vi "attck_din.vi"(9 "balls":T7[](array[typedef]), 10 "IA State":T1={"our_robots"=[], "enemy_robots"=[], "balls"=[], "geometry"={"field_length"=0, "field_width"=0, "goal_width"=0, "goal_depth"=0, "center_circle_radius"=0, "defense_width"=0, "defense_depth"=0, "free_kick_from_defense_dist"=0, "penalty_spot_from_field_line_dist"=0, "penalty_line_from_spot_dist"=0, "half_moon_depth"=0, "half_moon_width"=0}, "IA Judge"={"stage"="", "command"="", "our_goalie_id"=0.0, "enemy_goalie_id"=0.0, "command enum"=enum."Halt", "Time"=enum."Azul"}, "Received Timestamp"=timestamp(0 s since 1904-01-01), "Events"={"Touch"=FALSE, "id touch"=0.0, "Ball out of \nVision"=FALSE, "Ball inside \nGoalie area"=FALSE, "Robot not responding"=FALSE, "Robots responding status"=[1.0, 1.0, 1.0, 1.0, 1.0, 1.0], "Enemy Ball \nPossession"=FALSE, "Id ini Possession"=0.0, "Ball Possesion"=FALSE, "Id Possesion"=0.0, "Ball at\nour goal side"=FALSE, "Ball at\ntouchline"=FALSE, "Ball at\nenemy goal side"=FALSE}}, 11 "Robot in":T2) -> (3 "Robot out":T2)   [LabVIEW 2018]
uses:
  Core/AI Robot.ctl
  Functions Enum.ctl
  AttackerStates.ctl
  Path Planning/RRT/PathDests.ctl
  Path Planning/RRT/PathDest.ctl
  Core/AI Ball.ctl
  Core/AI Input.ctl
  Core/Field Size.ctl
  Core/AI Judge.ctl
  Command Enum.ctl
  Util/Events/Events.ctl
  <vilib>/Analysis/_algsub.llb/Real Vector Norm.vi
  <vilib>/Analysis/NI_AALPro.lvlib
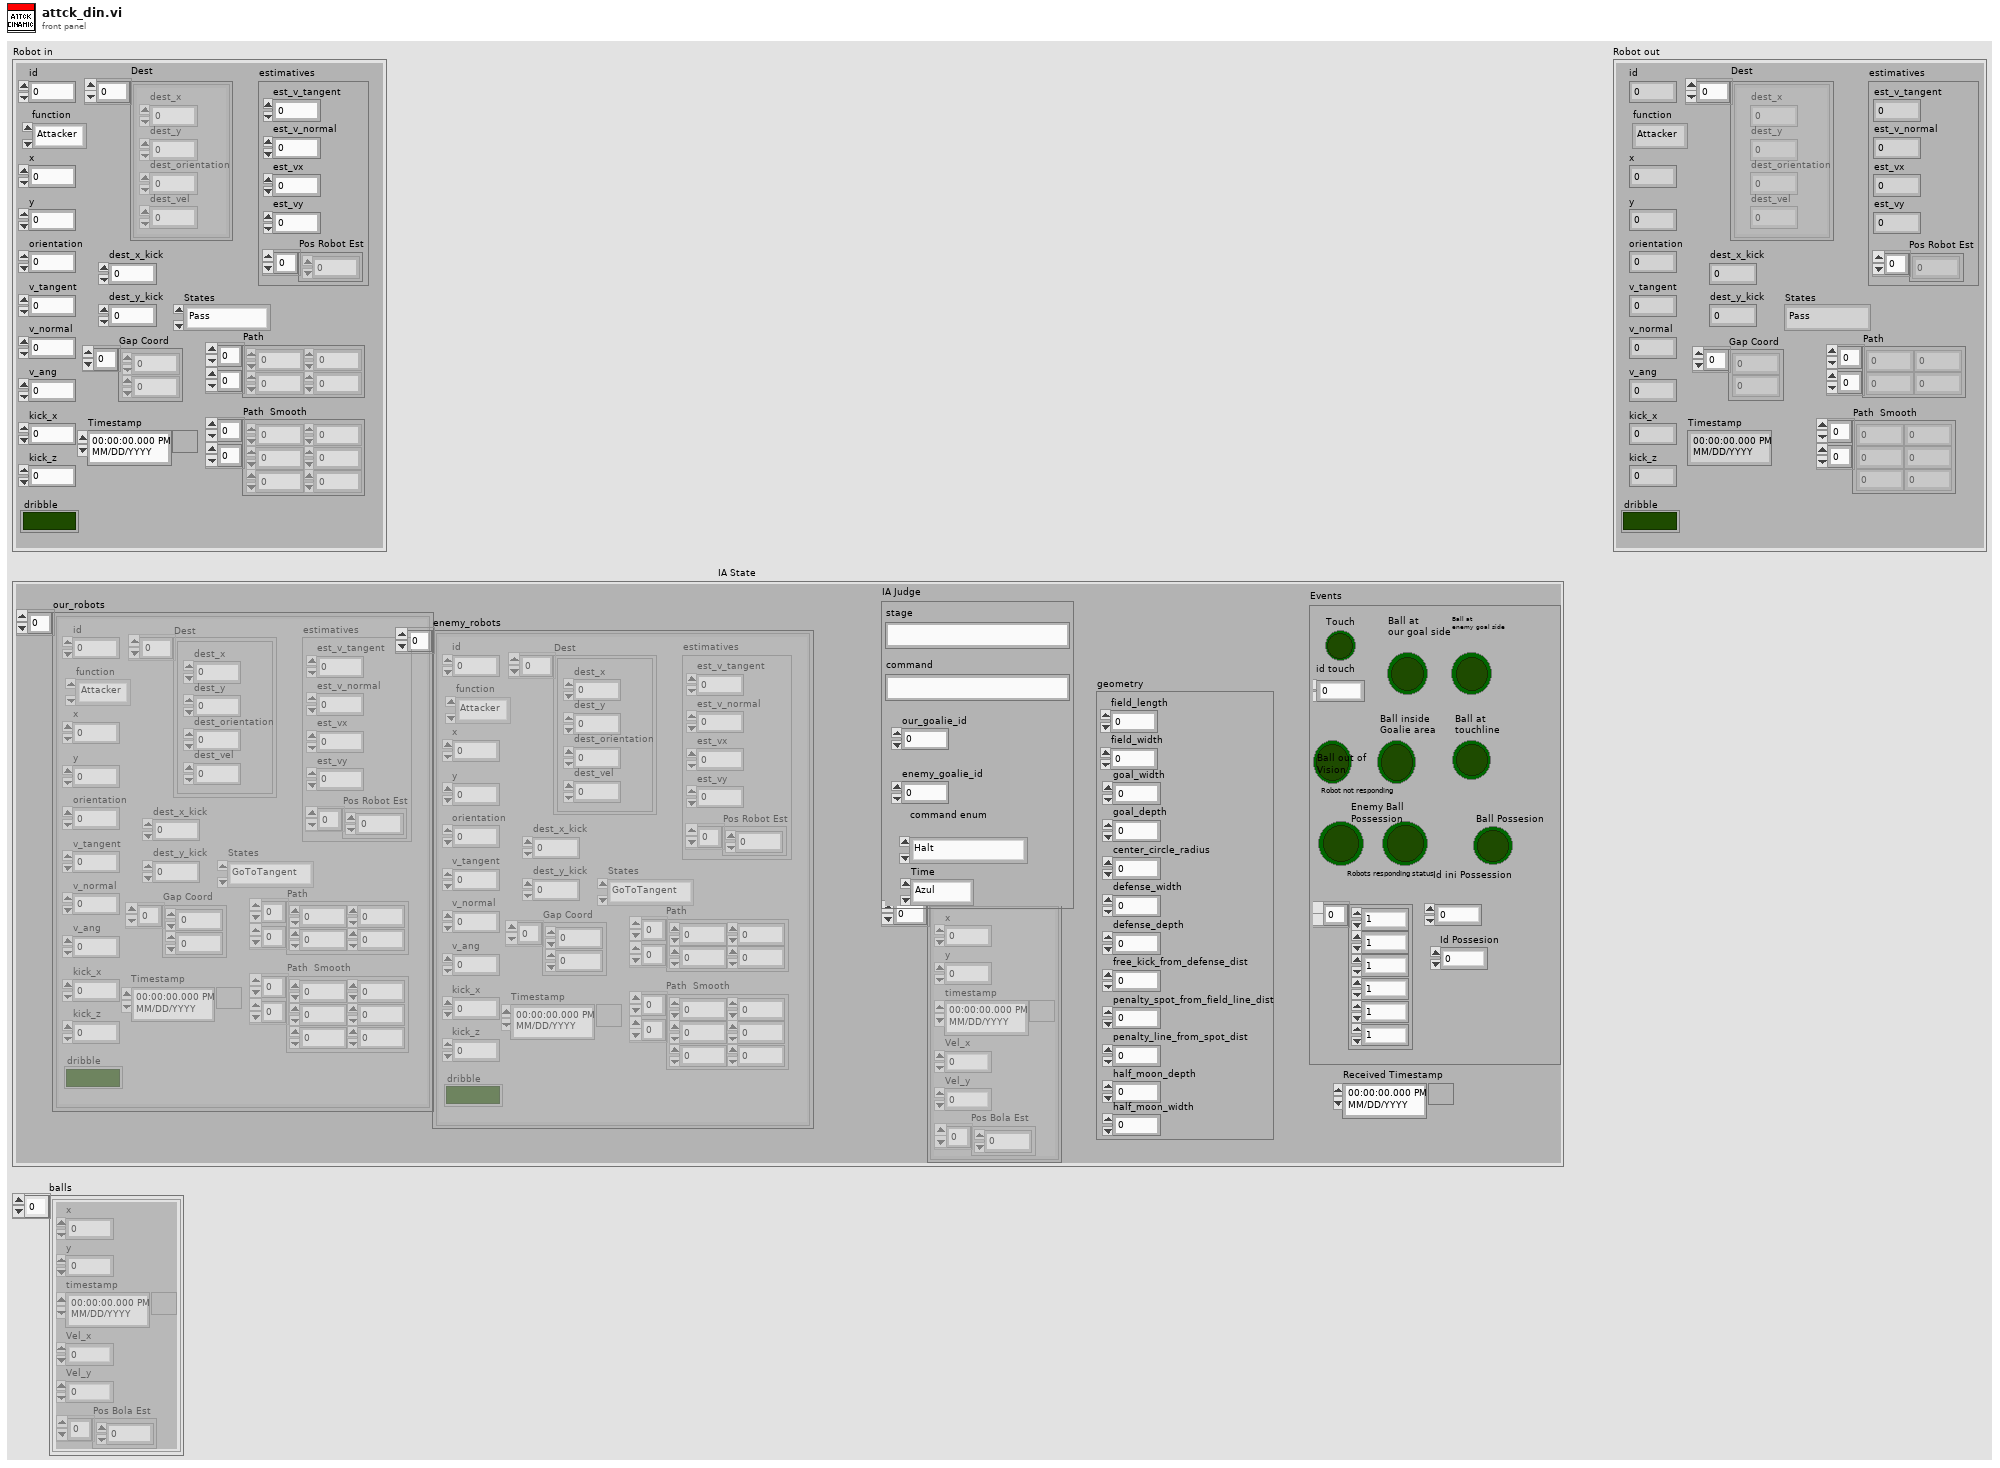
[diagram p1: front panel]
types:
  T1 = typedef "AI Input.ctl" = cluster{"our_robots":T2[], "enemy_robots":T2[], "balls":T7[], "geometry":T8, "IA Judge":T9, "Received Timestamp":timestamp, "Events":T11}
  T2 = typedef "AI Robot.ctl" = cluster{"id":u32, "function":T3, "x":dbl, "y":dbl, "orientation":dbl, "v_tangent":dbl, "v_normal":dbl, "v_ang":dbl, "kick_x":dbl, "kick_z":dbl, "dribble":bool, "Timestamp":timestamp, "estimatives":cluster{"est_v_tangent":dbl, "est_v_normal":dbl, "est_vx":dbl, "est_vy":dbl, "Pos Robot Est":dbl[]}, "dest_x_kick":dbl, "dest_y_kick":dbl, "Gap Coord":dbl[], "States":T4, "Path ":dbl[][], "Path  Smooth":dbl[][], "Dest":T5}
  T3 = typedef "Functions Enum.ctl" = enum16{"Attacker", "Goalie", "Defender", "Striker", "Goto 0", "Dummy", "Kicker", "ZigZag"}
  T4 = typedef "AttackerStates.ctl" = enum16{"Pass", "GoToTangent", "BallGetting", "GoToKick", "Rotate anti-clockwise", "Rotate Clockwise", ""}
  T5 = typedef "PathDests.ctl" = T6[]
  T6 = typedef "PathDest.ctl" = cluster{"dest_x":dbl, "dest_y":dbl, "dest_orientation":dbl, "dest_vel":dbl}
  T7 = typedef "AI Ball.ctl" = cluster{"x":dbl, "y":dbl, "timestamp":timestamp, "Vel_x":dbl, "Vel_y":dbl, "Pos Bola Est":dbl[]}
  T8 = typedef "Field Size.ctl" = cluster{"field_length":u32, "field_width":u32, "goal_width":u32, "goal_depth":u32, "center_circle_radius":u32, "defense_width":u32, "defense_depth":u32, "free_kick_from_defense_dist":u32, "penalty_spot_from_field_line_dist":u32, "penalty_line_from_spot_dist":u32, "half_moon_depth":u32, "half_moon_width":u32}
  T9 = typedef "AI Judge.ctl" = cluster{"stage":string, "command":string, "our_goalie_id":dbl, "enemy_goalie_id":dbl, "command enum":T10, "Time":enum16{"Azul", "Amarelo"}}
  T10 = typedef "Command Enum.ctl" = enum16{"Halt", "Stop", "Force Start", "PKA Normal Start", "Prepare Kickoff Ally", "PKE Normal Start", "Prepare Kickoff Enemy", "Prepare Penalty Ally", "PPA Normal Start", "Prepare Penalty Enemy", "PPE Normal Start", "Ball Placement Enemy Up", "Ball Placement Enemy Down", "Ball Placement Ally Up", "Ball Placement Ally Mid", "Ball Placement Ally Down", "Indirect Free Enemy", "Indirect Free Ally", "Timeout Enemy", "Timeout Ally", "Goal Enemy", "Goal Ally", "Normal Half Time", "Extra Time Break", "Extra Half Time", "None", "Post Game"}
  T11 = typedef "Events.ctl" = cluster{"Touch":bool, "id touch":dbl, "Ball out of \nVision":bool, "Ball inside \nGoalie area":bool, "Robot not responding":bool, "Robots responding status":dbl[], "Enemy Ball \nPossession":bool, "Id ini Possession":dbl, "Ball Possesion":bool, "Id Possesion":dbl, "Ball at\nour goal side":bool, "Ball at\ntouchline":bool, "Ball at\nenemy goal side":bool}
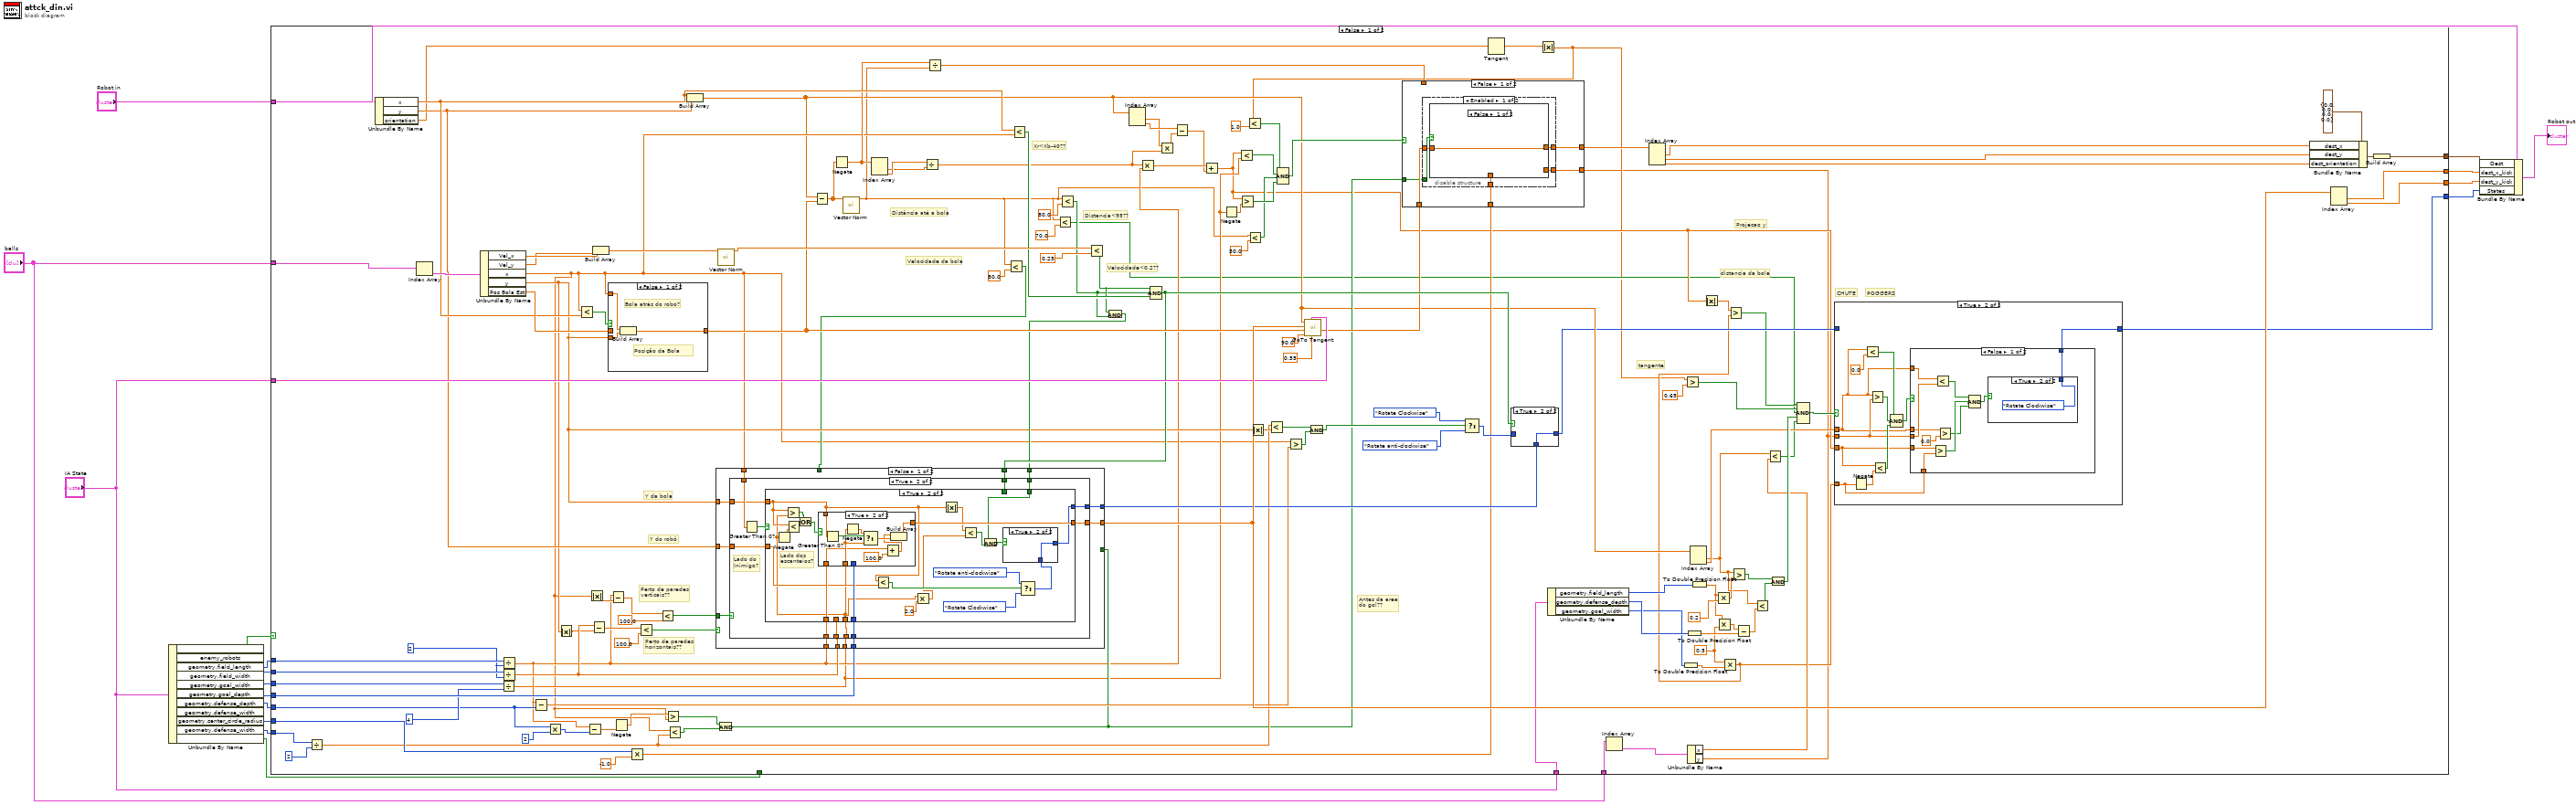
[diagram p0: block diagram]
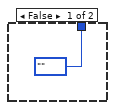
[diagram p3: hidden frame]
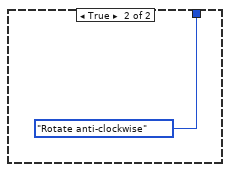
[diagram p4: hidden frame]
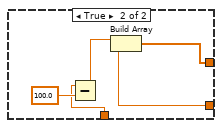
[diagram p5: hidden frame]
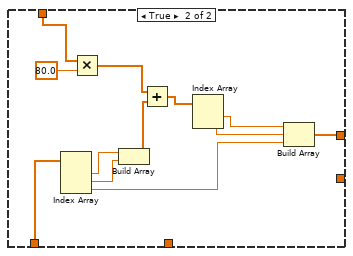
[diagram p7: hidden frame]
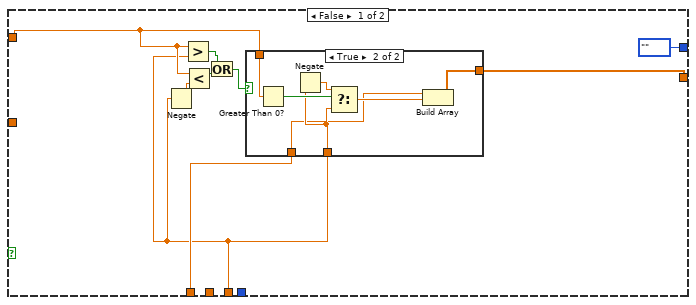
[diagram p10: hidden frame]
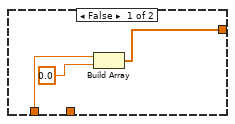
[diagram p11: hidden frame]
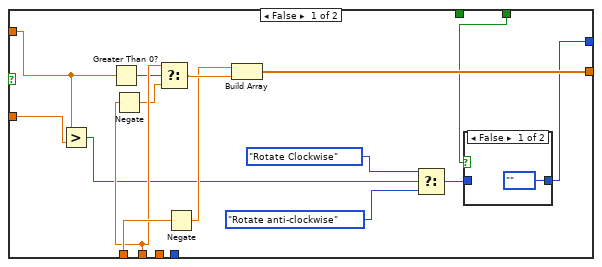
[diagram p12: hidden frame]
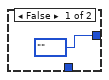
[diagram p14: hidden frame]
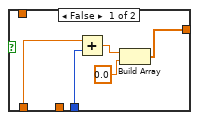
[diagram p15: hidden frame]
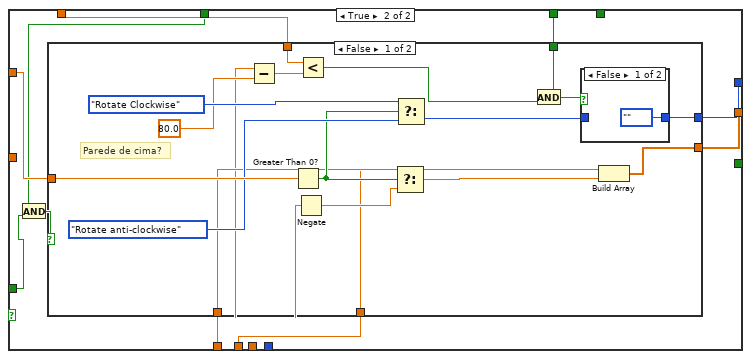
[diagram p16: hidden frame]
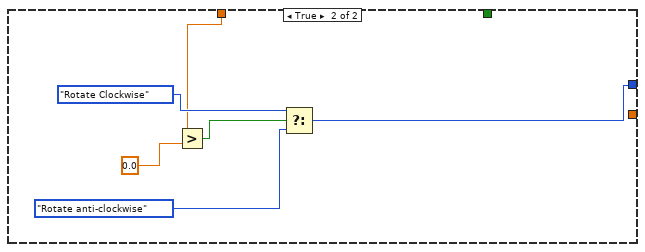
[diagram p18: hidden frame]
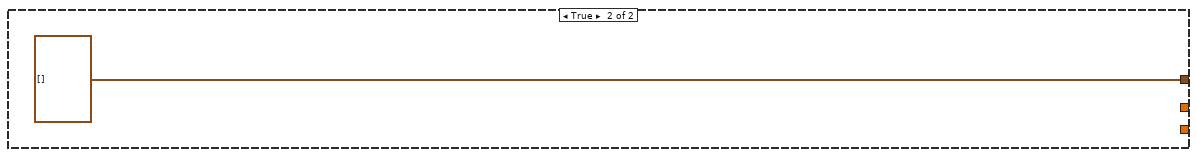
[diagram p19: hidden frame]
diagram:
  n1 = Unbundle By Name("IA State") -> ("Events.Ball out of \nVision"=w6:bool, "geometry.field_length"=w13:u32, "geometry.field_width"=w14:u32, "geometry.goal_width"=w15:u32, "geometry.goal_depth"=w9:u32, "geometry.defense_depth"=w7:u32, "geometry.center_circle_radius"=w4:u32, "geometry.defense_width"=w8:u32, "Events.Ball inside \nGoalie area"=w5:bool)  [unwired: 2 out]
  n2 = case shown="False" w6 {
    tunnel: [w151 _] -> w17
    tunnel: [w150 _] -> w16
    tunnel: w15 -> [w148 _]
    tunnel: "IA State" -> [w147 _]
    tunnel: w14 -> [w143 _]
    tunnel: w13 -> [w142 _]
    tunnel: "Robot in" -> [w141 _]
    tunnel: "balls" -> [w140 _]
    tunnel: [w137 T6[] []] -> w11
    tunnel: w9 -> [w136 _]
    tunnel: w8 -> [w135 _]
    tunnel: w7 -> [w96 _]
    tunnel: w5 -> [_ _]
    tunnel: w4 -> [w90 _]
    tunnel: "IA State" -> [w56 _]
    tunnel: "balls" -> [w58 _]
    tunnel: [w30 _] -> w1
    frame False {
      w36 = 0.5 ("y")
      w130 = u32 2 ("y")
      # "Y do robô"
      # "Y da bola"
      # "distancia da bola"
      # "tangente"
      # "Projecao y"
      # "POGGERS"
      # "CHUTE"
      # "Antes da area \ndo gol??"
      # "Perto de paredes \nverticais??"
      # "Perto de paredes \nhorizontais??"
      # "Velocidade<0,2??"
      # "Distancia<95??"
      # "Xr<Xb-40??"
      # "Velocidade da bola"
      # "Distância até a bola"
      n3 = Divide(x=w135, y=u32 2) -> (x/y=w86:dbl)
      n4 = Unbundle By Name(w141) -> ("x"=w113:dbl, "y"=w100:dbl, "orientation"=w51:dbl)
      n5 = Index Array(array=w140) -> (element=w133:T7)  [unwired: 1 in]
      n6 = Unbundle By Name(w133) -> ("Vel_x"=w123:dbl, "Vel_y"=w122:dbl, "x"=w59:dbl, "y"=w93:dbl, "Pos Bola Est"=w114:dbl[])
      n7 = Divide(x=w148, y=u32 4) -> (x/y=w67:dbl)
      n8 = Divide(x=w142, y=w130) -> (x/y=w75:dbl)
      n9 = Divide(x=w143, y=w130) -> (x/y=w117:dbl)
      n10 = Subtract(x=w75, y=w96) -> (x-y=w104:dbl)
      n11 = Multiply(x=w96, y=u32 2) -> (x*y=w95:u32)
      n12 = Absolute Value(x=w93) -> (abs(x)=w85:dbl)
      n13 = Less?(x=w59, y=w113) -> (x < y?=w116:bool)
      n14 = Subtract(x=w75, y=w95) -> (x-y=w94:dbl)
      n15 = Absolute Value(x=w59) -> (abs(x)=w129:dbl)
      n16 = Subtract(x=w117, y=w85) -> (x-y=w127:dbl)
      n17 = Build Array(w123, w122) -> (w121:dbl[])
      n18 = case shown="False" w116 {
        tunnel: [w209 w212] -> w115
        tunnel: w114 -> [_ w212]
        tunnel: w59 -> [w211 _]
        tunnel: w93 -> [w210 _]
        frame False {
          # "Bola atrás do robo?"
          # "Posição da Bola"
          n19 = Build Array(w211, w210) -> (w209:dbl[])
        }
        frame True {
          # "Posição futura da bola"
          # "Bola atrás do robo?"
        }
      }
      n20 = Subtract(x=w75, y=w129) -> (x-y=w128:dbl)
      n21 = Negate(x=w94) -> (-x=w92:dbl)
      n22 = Multiply(x=w90, y=-1.0) -> (x*y=w87:dbl)
      n23 = Less?(x=w127, y=100.0) -> (x < y?=w126:bool)
      n24 = Less?(x=w128, y=100.0) -> (x < y?=w125:bool)
      n25 = Greater?(x=w92, y=w59) -> (0:w83:bool)
      n26 = Less?(x=w59, y=w86) -> (x < y?=w84:bool)
      n27 = Build Array(w113, w100) -> (w53:dbl[])
      n28 = call-poly <vilib>:"Vector Norm.vi"("Input Vector"=w121) -> ("norm"=w119:dbl)  [unwired: 9 in, 1 out]
      n29 = And(x=w83, y=w84) -> (x .and. y?=w82:bool)
      n30 = Subtract(x=w53, y=w115) -> (x-y=w78:dbl[])
      n31 = Negate(x=w78) -> (-x=w61:dbl[])
      n32 = call-poly <vilib>:"Vector Norm.vi"("Input Vector"=w78) -> ("norm"=w22:dbl)  [unwired: 9 in, 1 out]
      n33 = Index Array(array=w61) -> (element #1=w76:dbl, element #2=w77:dbl)  [unwired: 2 in]
      n34 = Divide(x=w77, y=w76) -> (x/y=w71:dbl)
      n35 = Divide(x=w61, y=w22) -> (x/y=w60:dbl[])
      n36 = Less?(x=w22, y=80.0) -> (x < y?=w79:bool)
      n37 = Less?(x=w113, y=w59) -> (x < y?=w112:bool)
      n38 = Less?(x=w22, y=70.0) -> (x < y?=w23:bool)
      n39 = Less?(x=w22, y=80.0) -> (x < y?=w39:bool)
      n40 = Less?(x=w119, y=0.25) -> (x < y?=w99:bool)
      n41 = And(x=w99, y=w39) -> (x .and. y?=w98:bool)
      n42 = Index Array(array=w53) -> (element #1=w72:dbl, element #2=w74:dbl)  [unwired: 2 in]
      n43 = Multiply(x=w71, y=w75) -> (x*y=w73:dbl)
      n44 = Compound Arithmetic op=AND(w99, w39, w112) -> (w107:bool)
      n45 = case shown="False" w126 {
        tunnel: w93 -> [w222 w319]
        tunnel: w117 -> [w213 w313]
        tunnel: [w221 w318] -> w149
        tunnel: w125 -> [w224 w311]
        tunnel: w59 -> [w223 w315]
        tunnel: w75 -> [w220 w314]
        tunnel: w67 -> [w216 _]
        tunnel: w107 -> [w219 w316]
        tunnel: [w218 w317] -> w106
        tunnel: w136 -> [w217 _]
        tunnel: w100 -> [w215 _]
        tunnel: w98 -> [w214 _]
        tunnel: w82 -> [_ _]
        tunnel: w79 -> [_ w310]
        frame False {
          n46 = case shown="True" w224 {
            tunnel: w223 -> [_ w254]
            tunnel: w222 -> [w231 w253]
            tunnel: [w232 w252] -> w221
            tunnel: w220 -> [w233 w251]
            tunnel: w219 -> [_ w250]
            tunnel: [AttackerStates."" ("States") w249] -> w218
            tunnel: w217 -> [_ w248]
            tunnel: w213 -> [_ w247]
            tunnel: w216 -> [w229 w246]
            tunnel: w215 -> [_ w245]
            tunnel: w214 -> [_ w244]
            frame False {
              n47 = Negate(x=w229) -> (-x=w228:dbl)
              n48 = Greater?(x=w231, y=w229) -> (0:w225:bool)
              n49 = Less?(x=w231, y=w228) -> (x < y?=w226:bool)
              n50 = Or(x=w225, y=w226) -> (x .or. y?=w227:bool)
              n51 = case shown="True" w227 {
                tunnel: w233 -> [w235 w238]
                tunnel: [w236 w237] -> w232
                tunnel: w231 -> [_ w242]
                tunnel: w229 -> [_ w240]
                frame False {
                  n52 = Build Array(w235, 0.0 ("element")) -> (w236:dbl[])
                }
                frame True {
                  n53 = Greater Than 0?(x=w242) -> (x > 0?=w243:bool)
                  n54 = Negate(x=w240) -> (-x=w241:dbl)
                  n55 = Select(t=w241, s=w243, f=w240) -> (s? t:f=w239:dbl)
                  n56 = Build Array(w238, w239) -> (w237:dbl[])
                }
              }
            }
            frame True {
              # "Lado do\nInimigo?"
              n57 = Greater Than 0?(x=w254) -> (x > 0?=w255:bool)
              n58 = case shown="True" w255 {
                tunnel: w253 -> [w266 w284]
                tunnel: [w270 w288] -> w252
                tunnel: w251 -> [w268 w289]
                tunnel: w250 -> [_ _]
                tunnel: [w269 w279] -> w249
                tunnel: w248 -> [_ w287]
                tunnel: w247 -> [w267 _]
                tunnel: w246 -> [_ w274]
                tunnel: w245 -> [w265 w283]
                tunnel: w244 -> [w264 w276]
                frame False {
                  n59 = Greater?(x=w266, y=w265) -> (0:w256:bool)
                  n60 = Greater Than 0?(x=w266) -> (x > 0?=w259:bool)
                  n61 = Negate(x=w267) -> (-x=w263:dbl)
                  n62 = Select(t=w267, s=w259, f=w263) -> (s? t:f=w262:dbl)
                  n63 = Negate(x=w268) -> (-x=w261:dbl)
                  n64 = Build Array(w261, w262) -> (w270:dbl[])
                  n65 = Select(t=AttackerStates."Rotate Clockwise" ("States"), s=w256, f=AttackerStates."Rotate anti-clockwise" ("States")) -> (s? t:f=w257:T4)
                  n66 = case shown="False" w264 {
                    tunnel: [AttackerStates."" ("States") w272] -> w269
                    tunnel: w257 -> [_ w272]
                    frame False {
                    }
                    frame True {
                    }
                  }
                }
                frame True {
                  # "Lado dos\nescanteios?"
                  n67 = Negate(x=w274) -> (-x=w293:dbl)
                  n68 = Greater?(x=w284, y=w274) -> (0:w290:bool)
                  n69 = Less?(x=w284, y=w293) -> (x < y?=w291:bool)
                  n70 = Or(x=w290, y=w291) -> (x .or. y?=w292:bool)
                  n71 = case shown="True" w292 {
                    tunnel: w289 -> [w296 w301]
                    tunnel: [w299 w304] -> w288
                    tunnel: w284 -> [_ w308]
                    tunnel: w274 -> [_ w306]
                    tunnel: w287 -> [w297 _]
                    frame False {
                      n72 = Add(x=w296, y=w297) -> (x+y=w298:dbl)
                      n73 = Build Array(w298, 0.0 ("element")) -> (w299:dbl[])
                    }
                    frame True {
                      n74 = Greater Than 0?(x=w308) -> (x > 0?=w309:bool)
                      n75 = Negate(x=w306) -> (-x=w307:dbl)
                      n76 = Select(t=w307, s=w309, f=w306) -> (s? t:f=w305:dbl)
                      n77 = Add(x=w301, y=100.0) -> (x+y=w302:dbl)
                      n78 = Build Array(w302, w305) -> (w304:dbl[])
                    }
                  }
                  n79 = Less?(x=w284, y=w283) -> (x < y?=w282:bool)
                  n80 = Multiply(x=w274, y=2.0) -> (x*y=w273:dbl)
                  n81 = Absolute Value(x=w284) -> (abs(x)=w286:dbl)
                  n82 = Less?(x=w286, y=w273) -> (x < y?=w277:bool)
                  n83 = And(x=w276, y=w277) -> (x .and. y?=w278:bool)
                  n84 = Select(t=AttackerStates."Rotate anti-clockwise" ("States"), s=w282, f=AttackerStates."Rotate Clockwise" ("States")) -> (s? t:f=w285:T4)
                  n85 = case shown="True" w278 {
                    tunnel: w285 -> [_ w295]
                    tunnel: [AttackerStates."" ("States") w295] -> w279
                    frame False {
                    }
                    frame True {
                    }
                  }
                }
              }
            }
          }
        }
        frame True {
          n86 = And(x=w310, y=w311) -> (x .and. y?=w312:bool)
          n87 = case shown="False" w312 {
            tunnel: w319 -> [w336 _]
            tunnel: [w333 _] -> w318
            tunnel: [w330 w339] -> w317
            tunnel: w316 -> [w328 _]
            tunnel: w315 -> [w327 w340]
            tunnel: w314 -> [w321 _]
            tunnel: w313 -> [w320 _]
            frame False {
              # "Parede de cima?"
              n88 = Subtract(x=w320, y=80.0) -> (x-y=w326:dbl)
              n89 = Greater Than 0?(x=w336) -> (x > 0?=w329:bool)
              n90 = Negate(x=w320) -> (-x=w335:dbl)
              n91 = Less?(x=w327, y=w326) -> (x < y?=w323:bool)
              n92 = Select(t=w320, s=w329, f=w335) -> (s? t:f=w334:dbl)
              n93 = Select(t=AttackerStates."Rotate Clockwise" ("States"), s=w329, f=AttackerStates."Rotate anti-clockwise" ("States")) -> (s? t:f=w324:T4)
              n94 = And(x=w328, y=w323) -> (x .and. y?=w322:bool)
              n95 = case shown="False" w322 {
                tunnel: w324 -> [_ w338]
                tunnel: [AttackerStates."" ("States") w338] -> w330
                frame False {
                }
                frame True {
                }
              }
              n96 = Build Array(w321, w334) -> (w333:dbl[])
            }
            frame True {
              n97 = Greater?(x=w340, y=0.0) -> (0:w341:bool)
              n98 = Select(t=AttackerStates."Rotate Clockwise" ("States"), s=w341, f=AttackerStates."Rotate anti-clockwise" ("States")) -> (s? t:f=w339:T4)
            }
          }
        }
      }
      n99 = Multiply(x=w72, y=w71) -> (x*y=w70:dbl)
      n100 = Subtract(x=w74, y=w70) -> (x-y=w69:dbl)
      n101 = Add(x=w73, y=w69) -> (x+y=w28:dbl)
      n102 = Negate(x=w67) -> (-x=w68:dbl)
      n103 = Less?(x=w28, y=w67) -> (x < y?=w66:bool)
      n104 = Greater?(x=w28, y=w68) -> (0:w65:bool)
      n105 = Less?(x=w22, y=50.0) -> (x < y?=w63:bool)
      n106 = Absolute Value(x=w93) -> (abs(x)=w105:dbl)
      n107 = Less?(x=w86, y=w105) -> (x < y?=w103:bool)
      n108 = Greater?(x=w59, y=w104) -> (0:w102:bool)
      n109 = call "GoTo Tangent.vi"("Cone de chute"=0.55, "IA State Input in"=w147, "distance between ball and robot"=90.0, "Ball"=w115, "Target"=w149, "R"=w53) -> ("Destination"=w89:dbl[])  [unwired: 4 in, 1 out]
      n110 = And(x=w103, y=w102) -> (x .and. y?=w101:bool)
      n111 = Select(t=AttackerStates."Rotate Clockwise" ("States"), s=w101, f=AttackerStates."Rotate anti-clockwise" ("States")) -> (s? t:f=w108:T4)
      n112 = Tangent(1:w51) -> (0:w50:dbl)
      n113 = case shown="True" w107 {
        tunnel: [w207 w208] -> w31
        tunnel: w108 -> [_ _]
        tunnel: w106 -> [w207 w208]
        frame False {
        }
        frame True {
        }
      }
      n114 = Absolute Value(x=w50) -> (abs(x)=w21:dbl)
      n115 = Less?(x=w21, y=1.0) -> (x < y?=w19:bool)
      n116 = Compound Arithmetic op=AND(w19, w66, w63, w65) -> (w62:bool)
      n117 = Unbundle By Name(w56) -> ("geometry.field_length"=w54:u32, "geometry.defense_depth"=w46:u32, "geometry.goal_width"=w37:u32)
      n118 = Index Array(array=w58) -> (element=w57:T7)  [unwired: 1 in]
      n119 = To Double Precision Float(number=w37) -> (double precision float=w27:dbl)
      n120 = Greater?(x=w21, y=0.65) -> (0:w48:bool)
      n121 = To Double Precision Float(number=w46) -> (double precision float=w45:dbl)
      n122 = Unbundle By Name(w57) -> ("x"=w33:dbl, "y"=w18:dbl)
      n123 = case shown="False" w62 {
        tunnel: w89 -> [w182 w206]
        tunnel: [w181 w195] -> w88
        tunnel: w87 -> [w180 _]
        tunnel: w82 -> [w179 _]
        tunnel: w60 -> [_ w204]
        tunnel: w18 -> [w178 _]
        frame False {
          n124 = disable-structure shown="Enabled" {
            disable-tunnel: w182 -> [w187 w194]
            disable-tunnel: [w186 w194] -> w181
            disable-tunnel: w180 -> [w185 _]
            disable-tunnel: w179 -> [w184 _]
            disable-tunnel: w178 -> [w183 _]
            frame Enabled {
              n125 = case shown="False" w184 {
                tunnel: [w188 w193] -> w186
                tunnel: w187 -> [w188 _]
                tunnel: w185 -> [_ w190]
                tunnel: w183 -> [_ w189]
                frame False {
                }
                frame True {
                  n126 = Subtract(x=w190, y=100.0) -> (x-y=w191:dbl)
                  n127 = Build Array(w191, w189) -> (w193:dbl[])
                }
              }
            }
            frame Disabled {
            }
          }
        }
        frame True {
          n128 = Index Array(array=w206) -> (element #1=w201:dbl, element #2=w200:dbl, element #3=w196:dbl)  [unwired: 3 in]
          n129 = Multiply(x=w204, y=80.0) -> (x*y=w203:dbl[])
          n130 = Build Array(w201, w200) -> (w202:dbl[])
          n131 = Add(x=w203, y=w202) -> (x+y=w199:dbl[])
          n132 = Index Array(array=w199) -> (element #1=w198:dbl, element #2=w197:dbl)  [unwired: 2 in]
          n133 = Build Array(w198, w197, w196) -> (w195:dbl[])
        }
      }
      n134 = Index Array(array=w88) -> (element #1=w145:dbl, element #2=w146:dbl, element #3=w144:dbl)  [unwired: 3 in]
      n135 = Index Array(array=w53) -> (element #1=w32:dbl, element #2=w35:dbl)  [unwired: 2 in]
      n136 = To Double Precision Float(number=w54) -> (double precision float=w47:dbl)
      n137 = Absolute Value(x=w28) -> (abs(x)=w29:dbl)
      n138 = Multiply(x=w47, y=0.2) -> (x*y=w52:dbl)
      n139 = Multiply(x=w47, y=w36) -> (x*y=w44:dbl)
      n140 = Multiply(x=w36, y=w27) -> (x*y=w25:dbl)
      n141 = Greater?(x=w29, y=w25) -> (0:w26:bool)
      n142 = Greater?(x=w32, y=w52) -> (0:w41:bool)
      n143 = Subtract(x=w44, y=w45) -> (x-y=w43:dbl)
      n144 = Less?(x=w32, y=w43) -> (x < y?=w42:bool)
      n145 = Less?(x=w32, y=w33) -> (x < y?=w34:bool)
      n146 = And(x=w41, y=w42) -> (x .and. y?=w40:bool)
      n147 = Compound Arithmetic op=AND(w26, w48, w23, w40, w34) -> (w38:bool)
      n148 = case shown="True" w38 {
        tunnel: w28 -> [_ w153]
        tunnel: w35 -> [_ w155]
        tunnel: w25 -> [_ w160]
        tunnel: w18 -> [_ w159]
        tunnel: w31 -> [w152 _]
        tunnel: [w152 w158] -> w30
        frame False {
        }
        frame True {
          n149 = Negate(x=w160) -> (-x=w154:dbl)
          n150 = Less?(x=w155, y=0.0) -> (x < y?=w156:bool)
          n151 = Greater?(x=w155, y=w159) -> (0:w162:bool)
          n152 = Less?(x=w153, y=w154) -> (x < y?=w163:bool)
          n153 = Compound Arithmetic op=AND(w156, w162, w163) -> (w161:bool)
          n154 = case shown="False" w161 {
            tunnel: w160 -> [w169 _]
            tunnel: w153 -> [w170 _]
            tunnel: w159 -> [w171 _]
            tunnel: w155 -> [w174 _]
            tunnel: [w167 AttackerStates."Rotate anti-clockwise" ("States")] -> w158
            tunnel: w155 -> [w165 _]
            frame False {
              n155 = Greater?(x=w170, y=w169) -> (0:w172:bool)
              n156 = Less?(x=w174, y=w171) -> (x < y?=w173:bool)
              n157 = Greater?(x=w165, y=0.0) -> (0:w164:bool)
              n158 = Compound Arithmetic op=AND(w173, w172, w164) -> (w168:bool)
              n159 = case shown="True" w168 {
                tunnel: [AttackerStates."" ("States") AttackerStates."Rotate Clockwise" ("States")] -> w167
                frame False {
                }
                frame True {
                }
              }
            }
            frame True {
            }
          }
        }
      }
      n160 = Bundle By Name(cluster=T6 {"dest_x"=0.0, "dest_y"=0.0, "dest_orientation"=0.0, "dest_vel"=0.0} ("element"), "dest_x"=w145, "dest_y"=w146, "dest_orientation"=w144) -> (w138:T6)
      n161 = Index Array(array=w149) -> (element #1=w150:dbl, element #2=w151:dbl)  [unwired: 2 in]
      n162 = Build Array(w138) -> (w137:T6[])
    }
    frame True {
    }
  }
  n163 = Bundle By Name(cluster="Robot in", "Dest"=w11, "dest_x_kick"=w16, "dest_y_kick"=w17, "States"=w1) -> (→"Robot out":T2)
